vi "Fpga-OrderBook.vi"() -> ()   [LabVIEW 2016]
uses:
  <vilib>/Platform/TimedLoop/XDataNode/timing_clust.ctl
  <vilib>/Platform/TimedLoop/XDataNode/nitl_modes.ctl
  <vilib>/Platform/TimedLoop/XDataNode/wakeup.ctl
  <vilib>/rvi/Emulation/niFpgaSctlEmulationGetInTimedLoop.vi
  <vilib>/rvi/Emulation/niFpgaEmulationReportErrorSimple.vi
  <vilib>/rvi/Emulation/niFpgaGetClockAttributes.vi
  <vilib>/rvi/Emulation/niFpgaCriticalErrorInLSC.vi
  <vilib>/rvi/DataTransferAndStorage/Container/Common/niFpgaContainerGetUniqueNameForEmu.vi
  <vilib>/rvi/DataTransferAndStorage/Container/Common/niFpgaContainerSetEmuInfo.vi
  <vilib>/rvi/eio/common/nirviEmuReportErrorAndStop.vi
  <vilib>/rvi/Emulation/niFpgaEmulationIsFPGAContextNoSignature.vi
  <vilib>/rvi/errors/niFpgaSetErrorForExecOnDevCompSimple.vi
  <vilib>/rvi/FIFO/Fifo_Resource/nirvififoEmulationSetSize.vi
  <vilib>/rvi/FIFO/Fifo_Resource/nirviFifoEmulationQueueMgr.vi
  <instcachedir>/0/nirviFifoEmulationQueueMgr_E5CAEC123FF24DC58D834DCA3CDAA9B5.lvgen/nirviFifoEmulationQueueMgr_E5CAEC123FF24DC58D834DCA3CDAA9B5_011.vi
  <vilib>/rvi/FIFO/Fifo_Resource/nirvififoEmulationDetermineInputValidOut.vi
  <vilib>/rvi/FIFO/Fifo_Resource/nirvififoEmulationCreateLock.vi
  <vilib>/rvi/Emulation/niFpgaProcessEmulError.vi
  <vilib>/rvi/FIFO/Fifo_Resource/nirvififoEmulationObtainLock.vi
  <vilib>/rvi/FIFO/Fifo_Resource/nirvififoEmulationReleaseLock.vi
  <vilib>/rvi/occurrence/nirviWaitOnOccurrenceBase.vi
  <vilib>/rvi/errors/nirviReportUnexpectedCaseInternalError.vi
  <vilib>/rvi/errors/nirviReportUnexpectedCaseInternalError (U32).vi
  <vilib>/rvi/DataTransferAndStorage/Container/Common/niFpgaContainerExecOnDevCompGetState.vi
  <vilib>/rvi/Memory/Memory_Emulation/niFpgaMemoryEmulationCacheClearOnFirstRun.vi
  <vilib>/rvi/Memory/Memory_Emulation/nirvimemoryEmulationManagerCache_MakeExclusive.vi
  <vilib>/rvi/Memory/Memory_Emulation/niFpgaMemoryEmulationValidateCache.vi
  <vilib>/rvi/Memory/Memory_Emulation/nirvimemoryEmulationManagerCache_InsertValue.vi
  <vilib>/Utility/error.llb/Clear Errors.vi
  <vilib>/rvi/Memory/Memory_Emulation/nirvimemoryEmulationManagerCache_ReleaseExclusive.vi
  <vilib>/rvi/Memory/Memory_Emulation/nirvimemoryEmulationManagerCache_GetValue.vi
  <vilib>/rvi/Memory/Memory_Emulation/nirvimemoryEmulationManagerCache_SetValue.vi
  <vilib>/rvi/Emulation/niFpgaSctlEmulationResourceMgr.vi
  <instcachedir>/0/nirviFifoEmulationQueueMgr_E5CAEC123FF24DC58D834DCA3CDAA9B5.lvgen/nirviFifoEmulationQueueMgr_E5CAEC123FF24DC58D834DCA3CDAA9B5_010.vi
  <vilib>/Platform/TimedLoop/XDataNode/XDataNode.xnode
  <vilib>/rvi/LocalResourceManager/LocalResourceManager.xnode
  <vilib>/rvi/DataTransferAndStorage/Container/XNode/niFpgaContainer.xnode
  <vilib>/rvi/FIFO/Fifo_Resource/nirvififoEmulationWrite.vi
  <vilib>/rvi/Memory/Memory_Emulation/niFpgaMemoryEmulationRefIn.vi
  <vilib>/rvi/FIFO/Fifo_Resource/nirvififoEmulationRead.vi
  <vilib>/Platform/TimedLoop/XDataNode/XDNodeRunTimeDep.lvlib
panel:
  out "s? t:f 2":T1
  out "s? t:f":T1
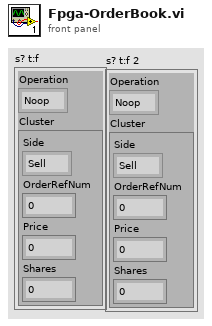
[diagram p1: front panel]
types:
  T1 = cluster{"Operation":enum16{"Noop", "GetAll", "AddOrder", "DeleteOrder"}, "Cluster":cluster{"Side":enum16{"Sell", "Buy"}, "OrderRefNum":u64, "Price":u32, "Shares":u32}}
  T2 = cluster{"Side":enum16{"Sell", "Buy"}, "OrderRefNum":u64, "Price":u32, "Shares":u32}
  T3 = typedef "XDNodeRunTimeDep.lvlib/timing_clust.ctl" = cluster{"Expected End [f-1]":u64, "Actual End [f-1]":u64, "Finished Late? [f-1]":bool, "Expected End [i-1]":u64, "Actual End [i-1]":u64, "Finished Late? [i-1]":bool, "Expected Start [i]":u64, "Actual Start [i]":u64, "Expected Start [f]":u64, "Actual Start [f]":u64, "Source Name":string, "Structure Name":string, "Period":i64, "Deadline":i64, "Offset":i64, "Start":i64, "Priority":i32, "Timeout":i32, "Mode":T4, "Wakeup Reason":T5, "Error":errorcluster, "Source Type":string, "Secondary Source Type":string, "Global End Time":u64, "Global Start Time":u64, "Frame Duration":u64, "Iteration Duration":u64, "Assigned CPU":i32, "I/O Scan Engine Mode":u32}
  T4 = typedef "XDNodeRunTimeDep.lvlib/nitl_modes.ctl" = enum32{"No Change", "Process missed periods, maintain original phase", "Discard missed periods, maintain original phase", "Process missed periods, ignore original phase", "Discard missed periods, ignore original phase"}
  T5 = typedef "XDNodeRunTimeDep.lvlib/wakeup.ctl" = enum32{"Normal", "Aborted", "Asynchronous wakeup", "Timing source error", "Timed loop error", "Timeout"}
  T6 = enum16{"Noop", "GetAll", "AddOrder", "DeleteOrder"}
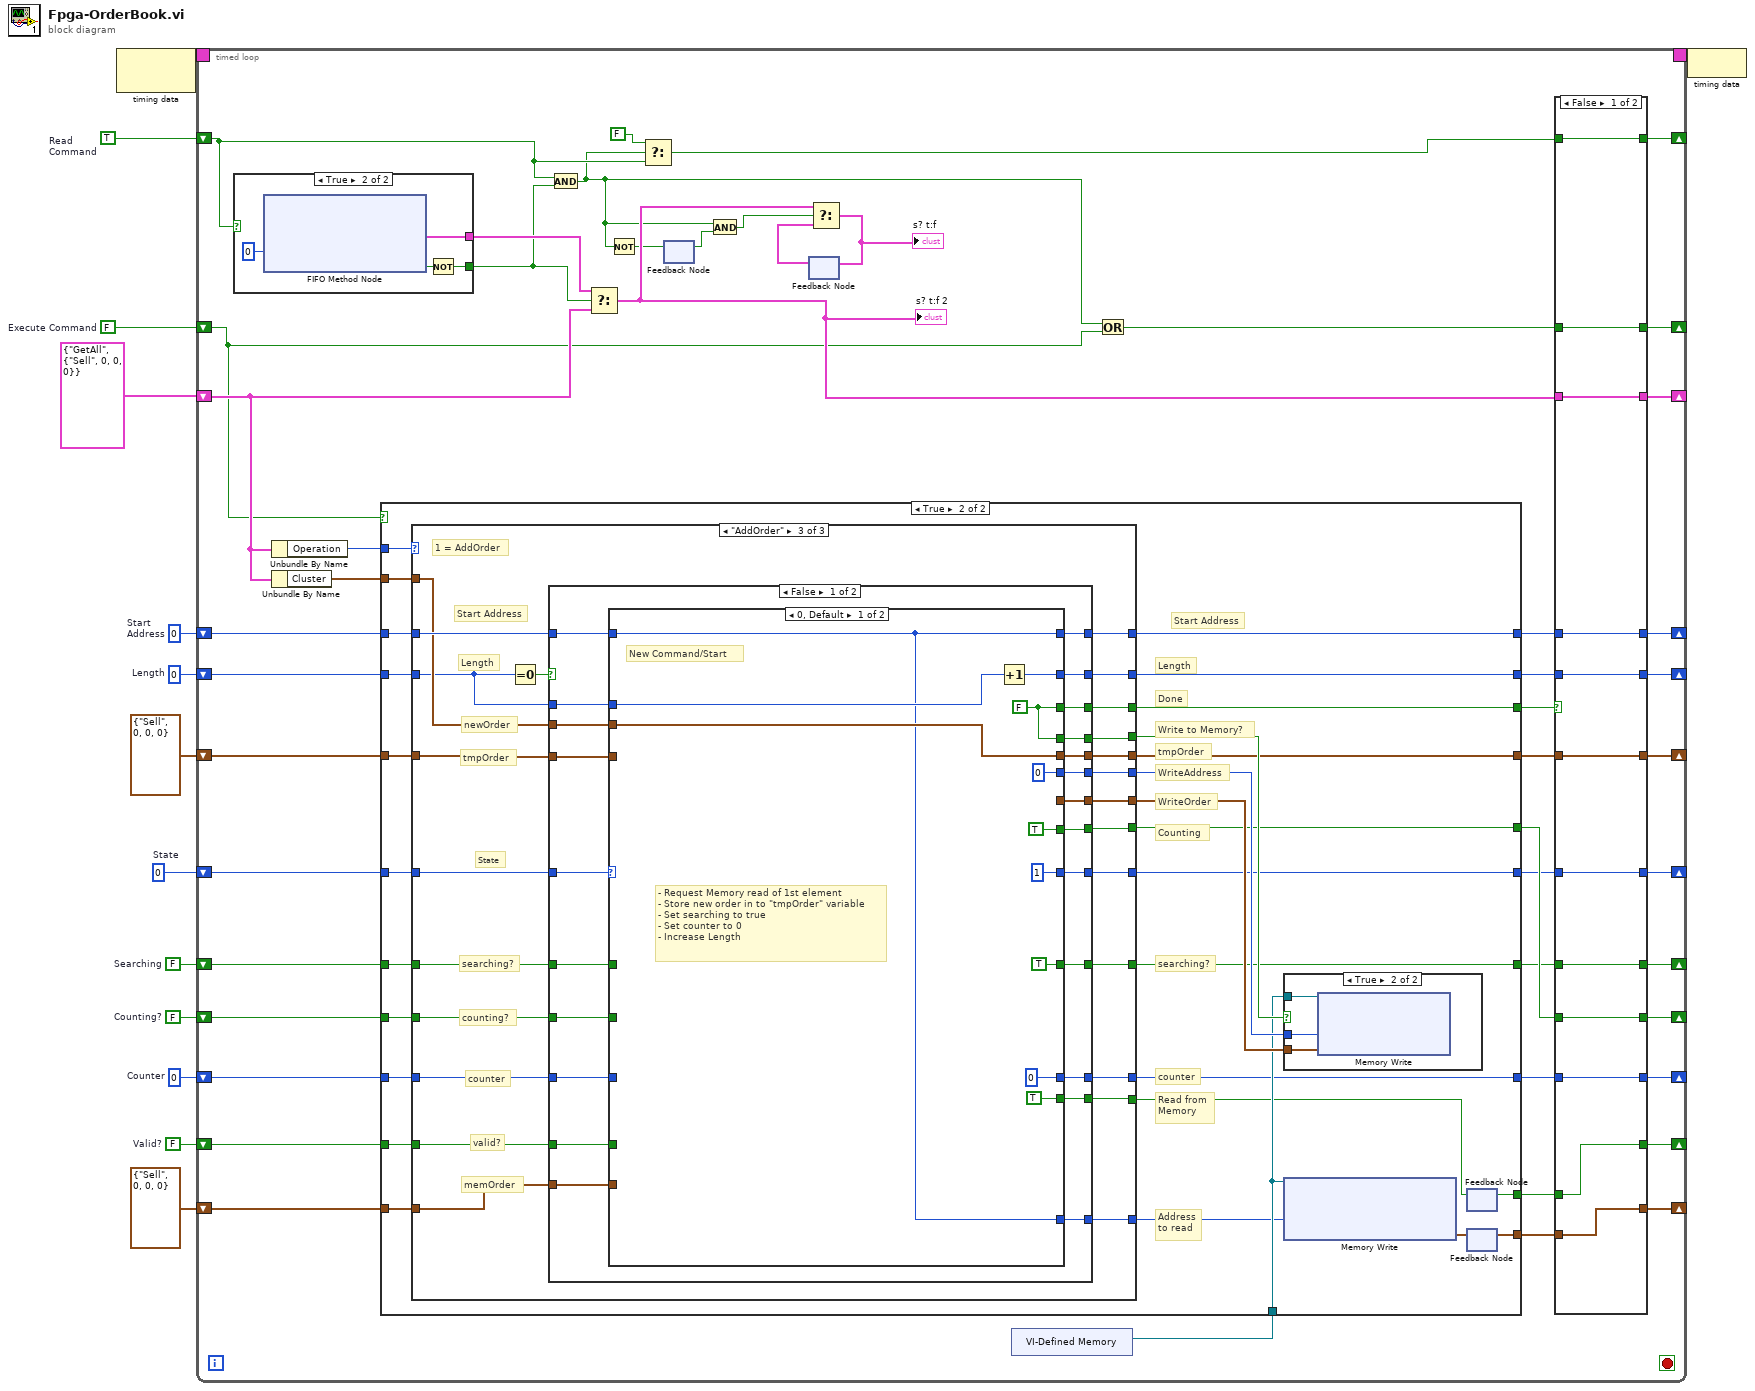
[diagram p0: block diagram]
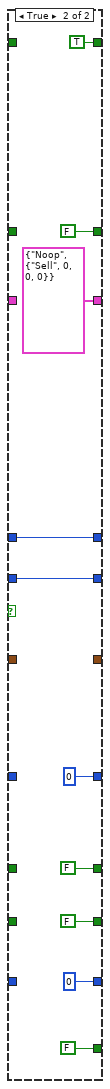
[diagram p2: hidden frame]
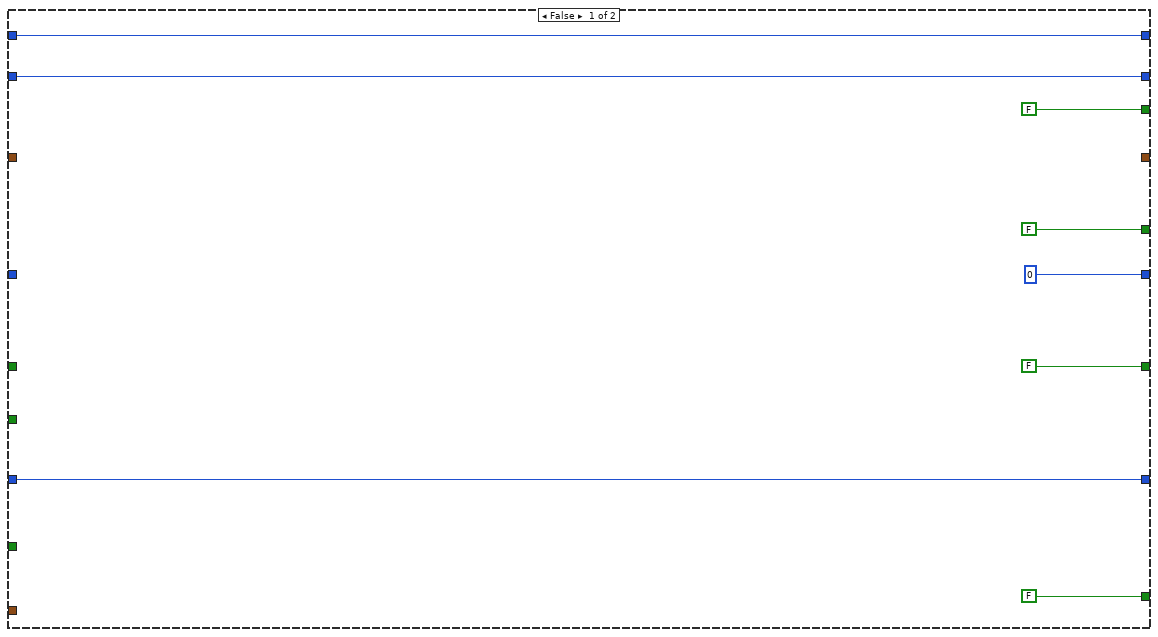
[diagram p3: hidden frame]
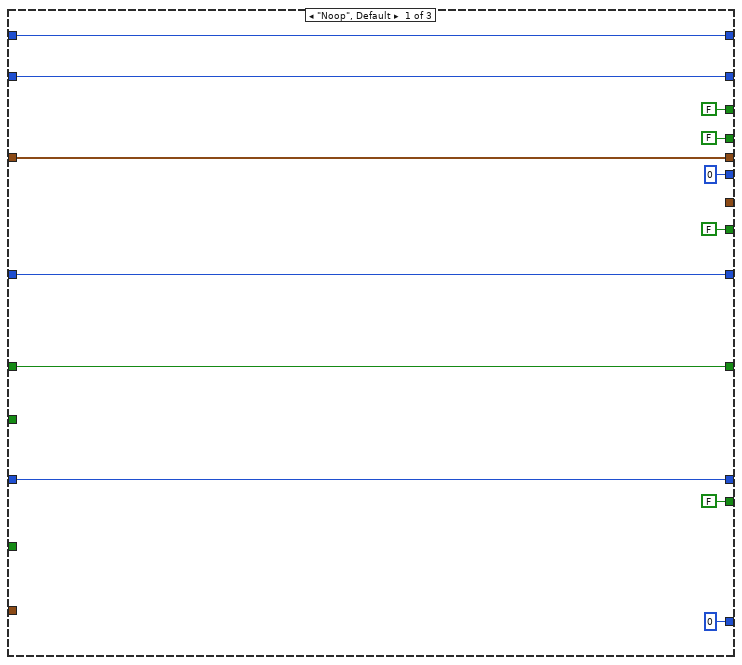
[diagram p5: hidden frame]
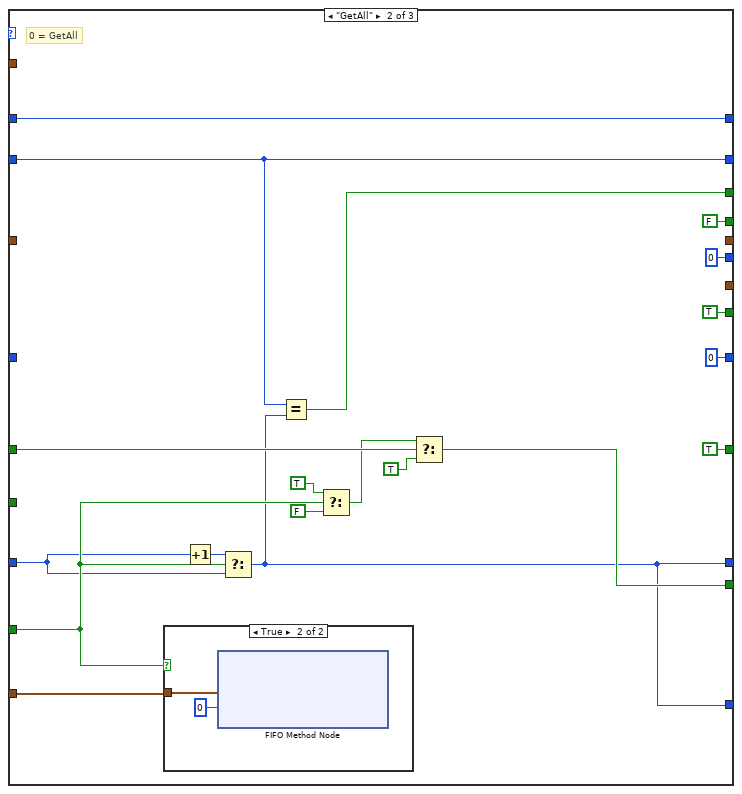
[diagram p6: hidden frame]
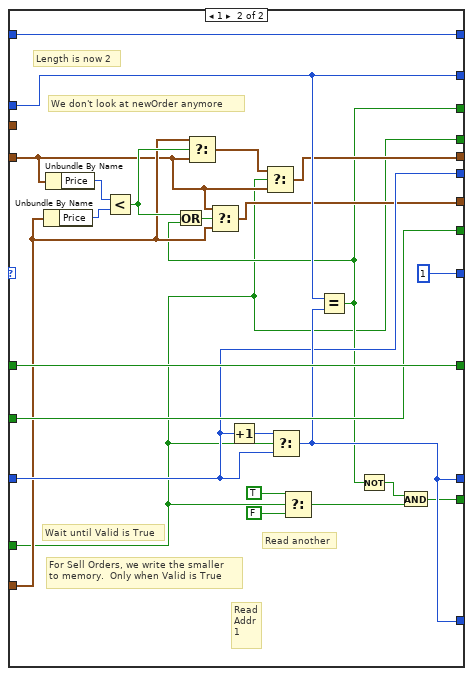
[diagram p8: hidden frame]
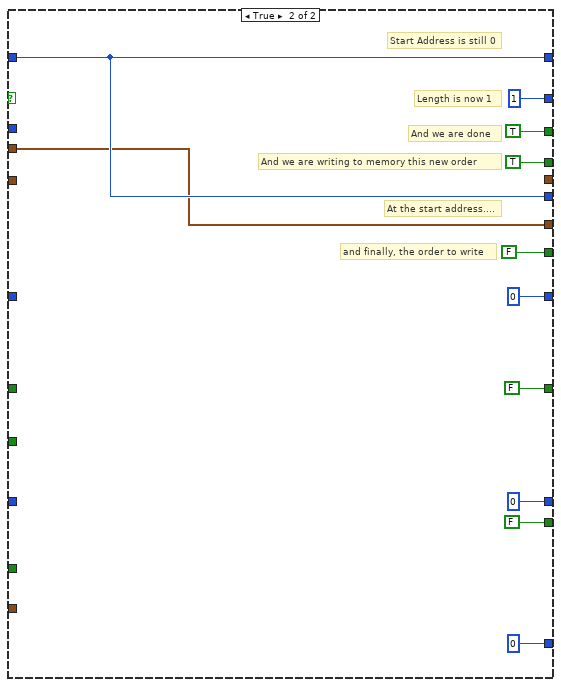
[diagram p9: hidden frame]
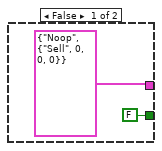
[diagram p10: hidden frame]
diagram:
  w4 = i16 0  # State
  w5 = FALSE  # Searching
  w6 = FALSE  # Valid?
  w7 = FALSE  # Counting?
  w8 = u64 0  # Counter
  w9 = FALSE  # Execute Command
  w11 = u64 0  # Length
  w10 = u64 0  # Start Address
  w12 = TRUE  # Read Command
  n1 = node-c288() -> (w14:T3)  [unwired: 1 in]
  n2 = timed-loop {
    timing: w14 -> [_]
    timing-out: [_] -> w13
    shift-right: [w31] -> _
    shift-left: w12 -> [w29]
    shift-right: [w39] -> _
    shift-left: w10 -> [w62]
    shift-right: [w37] -> _
    shift-left: w11 -> [w63]
    shift-right: [w26] -> _
    shift-left: w9 -> [w16]
    shift-right: [w50] -> _
    shift-left: w8 -> [w61]
    shift-right: [w53] -> _
    shift-left: w7 -> [w59]
    shift-right: [w45] -> _
    shift-left: T2 {"Side"=enum."Sell", "OrderRefNum"=0, "Price"=0, "Shares"=0} ("Cluster") -> [w57]
    shift-right: [w46] -> _
    shift-left: w6 -> [w58]
    shift-right: [w52] -> _
    shift-left: w5 -> [w56]
    shift-right: [w48] -> _
    shift-left: T2 {"Side"=enum."Sell", "OrderRefNum"=0, "Price"=0, "Shares"=0} ("Cluster") -> [w55]
    shift-right: [w42] -> _
    shift-left: w4 -> [w43]
    shift-right: [w35] -> _
    shift-left: T1 {"Operation"=enum."GetAll", "Cluster"={"Side"=enum."Sell", "OrderRefNum"=0, "Price"=0, "Shares"=0}} ("OrderBookCommand") -> [w28]
    stop <- _ stop-if-true
    n3 = case shown="True" w29 {
      tunnel: [FALSE ("Timed Out?") w253] -> w33
      tunnel: [T1 {"Operation"=enum."Noop", "Cluster"={"Side"=enum."Sell", "OrderRefNum"=0, "Price"=0, "Shares"=0}} ("Element") w254] -> w34
      frame False {
      }
      frame True {
        n4 = xnode ("FIFO Method Node")("Timeout"=0) -> ("Element"=w254:T1, "Timed Out?"=w255:bool)  [unwired: 1 in, 1 out]
        n5 = Not(x=w255) -> (.not. x?=w253:bool)
      }
    }
    n6 = Unbundle By Name(w28) -> ("Operation"=w15:T6)
    n7 = Unbundle By Name(w28) -> ("Cluster"=w27:T2)
    n8 = And(x=w29, y=w33) -> (x .and. y?=w21:bool)
    n9 = Select(t=w34, s=w33, f=w28) -> (s? t:f=w24:T1)
    "s? t:f 2" <- w24
    n10 = Not(x=w21) -> (.not. x?=w19:bool)
    n11 = Select(t=FALSE, s=w21, f=w29) -> (s? t:f=w30:bool)
    n12 = feedback-in #1(w19) -> ()
    n13 = feedback #1() -> (w18:bool)  [unwired: 1 in]
    n14 = And(x=w21, y=w18) -> (x .and. y?=w20:bool)
    n15 = feedback #2() -> (w22:T1)  [unwired: 1 in]
    n16 = Select(t=w24, s=w20, f=w22) -> (s? t:f=w23:T1)
    "s? t:f" <- w23
    n17 = feedback-in #2(w23) -> ()
    n18 = xnode "VI-Defined Memory"() -> ("Memory Out"=w60:refnum<k21>)
    n19 = case shown="True" w16 {
      tunnel: w15 -> [_ w121]
      tunnel: w63 -> [w93 w120]
      tunnel: [w93 w119] -> w36
      tunnel: w62 -> [w92 w117]
      tunnel: [w92 w118] -> w38
      tunnel: w61 -> [w90 w116]
      tunnel: [w90 w108] -> w49
      tunnel: [FALSE w115] -> w17
      tunnel: w60 -> [_ w109]
      tunnel: w27 -> [_ w104]
      tunnel: w59 -> [_ w111]
      tunnel: [FALSE w110] -> w54
      tunnel: [_ w95] -> w44
      tunnel: [FALSE w96] -> w40
      tunnel: w58 -> [_ w106]
      tunnel: w57 -> [_ w105]
      tunnel: w56 -> [_ w103]
      tunnel: [FALSE w102] -> w51
      tunnel: w55 -> [_ w100]
      tunnel: [_ w99] -> w47
      tunnel: w43 -> [_ w98]
      tunnel: [i16 0 ("State") w97] -> w41
      frame False {
      }
      frame True {
        # "tmpOrder"
        # "searching?"
        # "counter"
        # "Read from\nMemory"
        # "Address\nto read"
        # "Counting"
        # "WriteOrder"
        # "WriteAddress"
        # "Write to Memory?"
        # "Length"
        # "Start Address"
        # "Done"
        n20 = case shown="\"AddOrder\"" w121 {
          tunnel: w120 -> [w135 w141 w159]
          tunnel: [w135 w141 w181] -> w119
          tunnel: [w136 w155 w179] -> w118
          tunnel: w117 -> [w136 w155 w178]
          tunnel: w116 -> [w129 w139 w170]
          tunnel: [w129 w138 w169] -> w108
          tunnel: [FALSE w140 w177] -> w115
          tunnel: [FALSE ("Valid?") FALSE w176] -> w114
          tunnel: w104 -> [_ _ w174]
          tunnel: [_ _ w173] -> w113
          tunnel: [u64 0 ("Start\nAddress") u64 0 ("Start\nAddress") w175] -> w112
          tunnel: w111 -> [_ _ w172]
          tunnel: [FALSE ("Counting?") TRUE ("Counting?") w171] -> w110
          tunnel: [FALSE ("f") w142 w165] -> w94
          tunnel: w106 -> [_ w148 w164]
          tunnel: w105 -> [_ w137 w163]
          tunnel: w103 -> [w130 w145 w168]
          tunnel: [w130 TRUE w167] -> w102
          tunnel: [u64 0 ("Counter") w138 w166] -> w101
          tunnel: w100 -> [w134 _ w162]
          tunnel: [w134 _ w161] -> w99
          tunnel: w98 -> [w131 _ w160]
          tunnel: [w131 i16 0 ("State") w158] -> w97
          frame "Noop", Default {
          }
          frame "GetAll" {
            # "0 = GetAll"
            n21 = case shown="True" w148 {
              tunnel: w137 -> [_ w156]
              frame False {
              }
              frame True {
                n22 = xnode ("FIFO Method Node")("Element"=w156, "Timeout"=0) -> ()  [unwired: 1 in, 2 out]
              }
            }
            n23 = Increment(x=w139) -> (x+1=w149:u64)
            n24 = Select(t=w149, s=w148, f=w139) -> (s? t:f=w138:u64)
            n25 = Equal?(x=w141, y=w138) -> (x = y?=w140:bool)
            n26 = Select(t=TRUE, s=w148, f=FALSE) -> (s? t:f=w144:bool)
            n27 = Select(t=w144, s=w145, f=TRUE) -> (s? t:f=w142:bool)
          }
          frame "AddOrder" {
            # "State"
            # "Length"
            # "Start Address"
            # "memOrder"
            # "valid?"
            # "counter"
            # "counting?"
            # "searching?"
            # "tmpOrder"
            # "newOrder"
            # "1 = AddOrder"
            n28 = Equal To 0?(x=w159) -> (x = 0?=w180:bool)
            n29 = case shown="False" w180 {
              tunnel: [w203 u64 1 ("t")] -> w181
              tunnel: [w192 w247] -> w179
              tunnel: w178 -> [w191 w247]
              tunnel: [w199 TRUE] -> w177
              tunnel: [w198 TRUE] -> w176
              tunnel: [w197 w247] -> w175
              tunnel: w174 -> [w200 w246]
              tunnel: [w201 w246] -> w173
              tunnel: w172 -> [w182 _]
              tunnel: [w195 FALSE] -> w171
              tunnel: w170 -> [w184 _]
              tunnel: [w189 u64 0] -> w169
              tunnel: w168 -> [w183 _]
              tunnel: [w194 FALSE] -> w167
              tunnel: [w190 u64 0] -> w166
              tunnel: [w193 FALSE] -> w165
              tunnel: w164 -> [w187 _]
              tunnel: w163 -> [w185 _]
              tunnel: w162 -> [w186 _]
              tunnel: [w196 _] -> w161
              tunnel: w160 -> [w204 _]
              tunnel: w159 -> [w202 _]
              tunnel: [w188 i16 0 ("State")] -> w158
              frame False {
                n30 = case shown="0, Default" w204 {
                  tunnel: [w205 w230] -> w203
                  tunnel: w202 -> [w215 w230]
                  tunnel: [_ w226] -> w201
                  tunnel: w200 -> [w212 _]
                  tunnel: [w214 w218] -> w199
                  tunnel: [w214 w216] -> w198
                  tunnel: [u64 0 ("Start\nAddress") w229] -> w197
                  tunnel: [w212 w225] -> w196
                  tunnel: [TRUE w237] -> w195
                  tunnel: [TRUE w238] -> w194
                  tunnel: [TRUE w219] -> w193
                  tunnel: [w208 w239] -> w192
                  tunnel: w191 -> [w208 w239]
                  tunnel: [w208 w231] -> w190
                  tunnel: [u64 0 w231] -> w189
                  tunnel: [i16 1 ("State") i16 1 ("State")] -> w188
                  tunnel: w187 -> [_ w216]
                  tunnel: w186 -> [_ w220]
                  tunnel: w185 -> [_ w221]
                  tunnel: w184 -> [_ w229]
                  tunnel: w183 -> [_ w238]
                  tunnel: w182 -> [_ w237]
                  frame 0, Default {
                    w214 = FALSE
                    # "- Request Memory read of 1st element\n- Store new order in to \"tmpOrder\" variable\n- Set searching to true\n- Set counter to 0\n- Increase Length"
                    # "New Command/Start"
                    n31 = Increment(x=w215) -> (x+1=w205:u64)
                  }
                  frame 1 {
                    # "Read\nAddr\n1"
                    # "Read another"
                    # "Wait until Valid is True"
                    # "For Sell Orders, we write the smaller\nto memory.  Only when Valid is True"
                    # "We don't look at newOrder anymore"
                    # "Length is now 2"
                    n32 = Unbundle By Name(w221) -> ("Price"=w227:u32)
                    n33 = Unbundle By Name(w220) -> ("Price"=w228:u32)
                    n34 = Less?(x=w228, y=w227) -> (x < y?=w223:bool)
                    n35 = Select(t=w221, s=w223, f=w220) -> (s? t:f=w224:T2)
                    n36 = Increment(x=w229) -> (x+1=w233:u64)
                    n37 = Select(t=w224, s=w216, f=w220) -> (s? t:f=w225:T2)
                    n38 = Select(t=w233, s=w216, f=w229) -> (s? t:f=w231:u64)
                    n39 = Select(t=TRUE, s=w216, f=FALSE) -> (s? t:f=w236:bool)
                    n40 = Equal?(x=w230, y=w231) -> (x = y?=w218:bool)
                    n41 = Or(x=w223, y=w218) -> (x .or. y?=w222:bool)
                    n42 = Select(t=w220, s=w222, f=w221) -> (s? t:f=w226:T2)
                    n43 = Not(x=w218) -> (.not. x?=w217:bool)
                    n44 = And(x=w217, y=w236) -> (x .and. y?=w219:bool)
                  }
                }
              }
              frame True {
                # "and finally, the order to write"
                # "At the start address...."
                # "And we are writing to memory this new order"
                # "And we are done"
                # "Length is now 1"
                # "Start Address is still 0"
              }
            }
          }
        }
        n45 = case shown="True" w114 {
          tunnel: w109 -> [_ w124]
          tunnel: w113 -> [_ w122]
          tunnel: w112 -> [_ w123]
          frame False {
          }
          frame True {
            n46 = xnode ("Memory Write")("Address"=w123, "Data"=w122, "Memory In"=w124) -> ()  [unwired: 1 out]
          }
        }
        n47 = xnode ("Memory Write")("Address"=w101, "Memory In"=w109) -> ("Data"=w107:T2)  [unwired: 1 out]
        n48 = feedback-in #3(w94) -> ()
        n49 = feedback #3() -> (w96:bool)  [unwired: 1 in]
        n50 = feedback-in #4(w107) -> ()
        n51 = feedback #4() -> (w95:T2)  [unwired: 1 in]
      }
    }
    n52 = Or(x=w21, y=w16) -> (x .or. y?=w25:bool)
    n53 = case shown="False" w17 {
      tunnel: w54 -> [w75 _]
      tunnel: [w75 FALSE ("Counting?")] -> w53
      tunnel: [w74 FALSE] -> w52
      tunnel: w51 -> [w74 _]
      tunnel: [w73 u64 0 ("Counter")] -> w50
      tunnel: w49 -> [w73 _]
      tunnel: [w72 _] -> w48
      tunnel: w47 -> [w72 _]
      tunnel: [w71 FALSE] -> w46
      tunnel: w40 -> [w71 _]
      tunnel: [w70 _] -> w45
      tunnel: w44 -> [w70 _]
      tunnel: [w69 i16 0 ("State")] -> w42
      tunnel: w41 -> [w69 _]
      tunnel: [w68 w77] -> w39
      tunnel: w38 -> [w68 w77]
      tunnel: [w67 w76] -> w37
      tunnel: w36 -> [w67 w76]
      tunnel: w24 -> [w66 _]
      tunnel: [w66 T1 {"Operation"=enum."Noop", "Cluster"={"Side"=enum."Sell", "OrderRefNum"=0, "Price"=0, "Shares"=0}} ("Element")] -> w35
      tunnel: [w65 TRUE] -> w31
      tunnel: w30 -> [w65 _]
      tunnel: [w64 FALSE] -> w26
      tunnel: w25 -> [w64 _]
      frame False {
      }
      frame True {
      }
    }
  }
  n54 = node-c288(w13) -> ()
